vi "Wait-for-lasing-end.vi"(8 "error in (no error)":errorcluster, 11 "Object ref in":T1) -> (0 "error out":errorcluster, 1 "Succes?":bool, 3 "Object ref out":T1)   [LabVIEW 2013, in "SLMControl.lvlib" / "SC-Main.lvclass"]
uses:
  SC-Main.lvclass
  Object-reference.ctl
  UI/Control-names.ctl
  SC-Main.lvclass/SC-Main.ctl
  Read Lasing control.vi
  Read UI.vi
  UI/Set-control-boolean.vi
  UI/Set-control-string.vi
  UI/Set-control-double.vi
  SM1000/SM1000.lvclass
  UI/SC-UI.lvclass
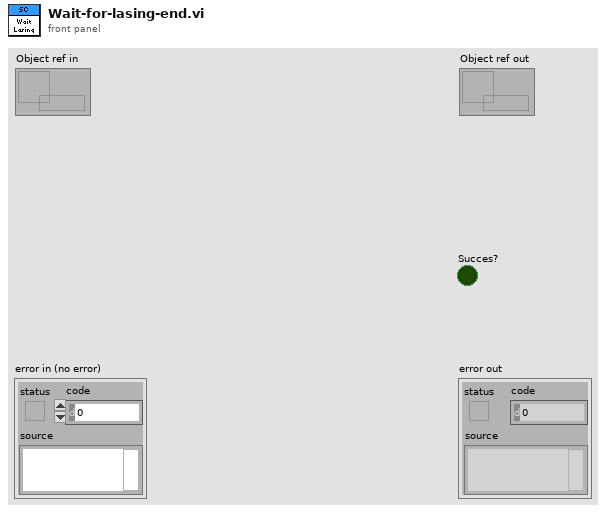
[diagram p1: front panel]
types:
  T1 = typedef "SLMControl.lvlib/SC-Main.lvclass/Object-reference.ctl" = refnum<data-value>
  T2 = typedef "SLMControl.lvlib/SC-UI.lvclass/Control-names.ctl" = enum16{"Com-in", "Com-out", "Help", "Status", "Load configuration", "Save configuration", "Load lasing files", "Load deposition files", "Clear", "Files", "Activate", "Execute", "Abort", "Options", "Current layer", "Current iteration", "Last elapsed time", "Deposition status", "Lasing job", "Status LEDs", "Exiting led", "Initialized led", "Files loaded led", "Activated led", "Executing led", "Deposition led", "Lasing job led", "Lasing led"}
  T3 = typedef "SLMControl.lvlib/SM1000.lvclass/Object-reference.ctl" = refnum<data-value>
  T4 = typedef "SLMControl.lvlib/SC-UI.lvclass/Panes-reference.ctl" = refnum<data-value>
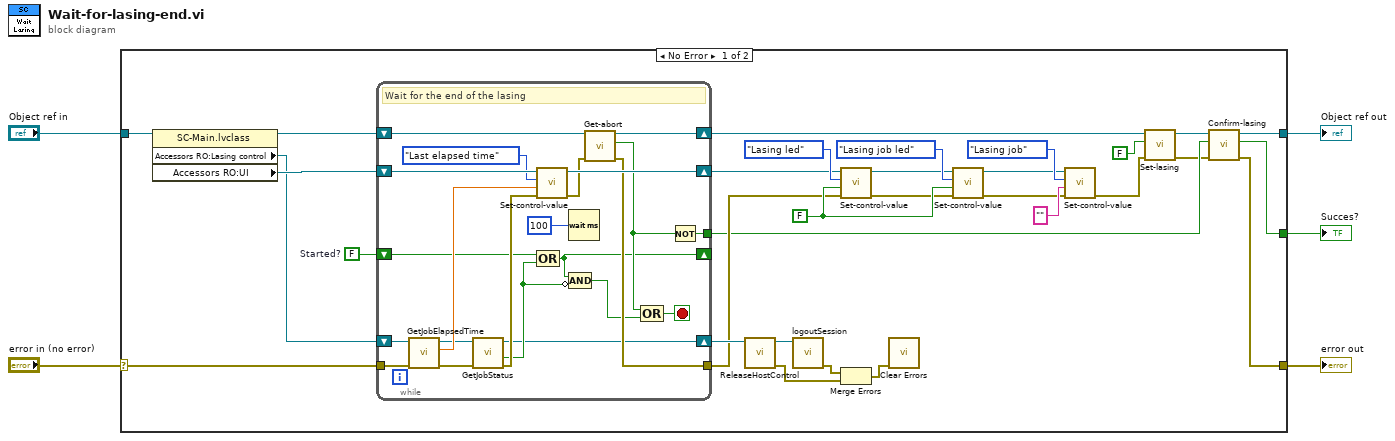
[diagram p0: block diagram]
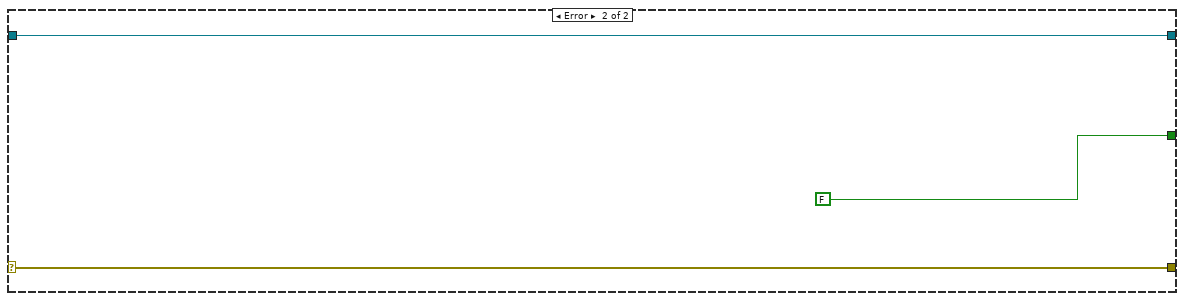
[diagram p2: hidden frame]
diagram:
  n1 = case shown="No Error" "error in (no error)" {
    selector: "error in (no error)" -> [w19 w61]
    tunnel: [w7 w61] -> w4
    tunnel: [w10 w60] -> w2
    tunnel: "Object ref in" -> [w36 w60]
    tunnel: [w9 FALSE] -> w1
    frame No Error {
      w12 = FALSE  # Started?
      w27 = FALSE
      n2 = property class="SC-Main.lvclass"(reference=w36) -> (reference out=w35:T1, "Accessors RO:Lasing control"=w13:T3, "Accessors RO:UI"=w34:T4)  [unwired: 1 in, 1 out]
      n3 = while {
        shift-right: [w51] -> w23
        shift-left: w35 -> [w58]
        tunnel: [w56] -> w8
        shift-right: [w40] -> w20
        shift-left: w13 -> [w39]
        tunnel: [w49] -> w18
        shift-right: [w54] -> w30
        shift-left: w34 -> [w55]
        tunnel: w19 -> [w38]
        shift-right: [w42] -> _
        shift-left: w12 -> [w44]
        stop <- w57 stop-if-true
        # "Wait for the end of the lasing"
        n4 = call "GetJobElapsedTime.vi"("error in (no error)"=w38, "SM1000-control in"=w39) -> ("error out"=w46:errorcluster, "Elapsed time"=w52:dbl, "SM1000-control out"=w37:T3)  [unwired: 7 in]
        n5 = call "GetJobStatus.vi"("error in (no error)"=w46, "SM1000-control in"=w37) -> ("error out"=w45:errorcluster, "Busy?"=w43:bool, "SM1000-control out"=w40:T3)  [unwired: 7 in]
        n6 = call-poly "Set-control-value.vi"("error in (no error)"=w45, "Value"=w52, "Control name"=Control-names."Last elapsed time", "Panes in"=w55) -> ("error out"=w50:errorcluster, "Panes out"=w54:T4)  [unwired: 6 in]
        n7 = Compound Arithmetic op=OR(w44, w43) -> (w42:bool)
        n8 = Wait (ms)(milliseconds to wait=u32 100) -> ()  [unwired: 1 out]
        n9 = Compound Arithmetic op=AND(w42, invert w43) -> (w41:bool)
        n10 = call "Get-abort.vi"("error in (no error)"=w50, "Object ref in"=w58) -> ("error out"=w49:errorcluster, "Abort"=w48:bool, "Object ref out"=w51:T1)  [unwired: 7 in]
        n11 = Compound Arithmetic op=OR(w48, w41) -> (w57:bool)
        n12 = Not(x=w48) -> (.not. x?=w56:bool)
      }
      n13 = call "ReleaseHostControl.vi"("SM1000-control in"=w20) -> ("error out"=w15:errorcluster, "SM1000-control out"=w17:T3)  [unwired: 9 in]
      n14 = call "logoutSession.vi"("SM1000-control in"=w17) -> ("error out"=w16:errorcluster)  [unwired: 9 in, 1 out]
      n15 = call-poly "Set-control-value.vi"("error in (no error)"=w18, "Value"=w27, "Control name"=Control-names."Lasing led", "Panes in"=w30) -> ("error out"=w25:errorcluster, "Panes out"=w29:T4)  [unwired: 6 in]
      n16 = Merge Errors(w16, w15) -> (w14:errorcluster)
      n17 = call <vilib>:"Clear Errors.vi"("error in (no error)"=w14) -> ()  [unwired: 6 in, 1 out]
      n18 = call-poly "Set-control-value.vi"("error in (no error)"=w25, "Value"=w27, "Control name"=Control-names."Lasing job led", "Panes in"=w29) -> ("error out"=w24:errorcluster, "Panes out"=w28:T4)  [unwired: 6 in]
      n19 = call-poly "Set-control-value.vi"("error in (no error)"=w24, "Value"="", "Control name"=Control-names."Lasing job", "Panes in"=w28) -> ("error out"=w22:errorcluster)  [unwired: 6 in, 1 out]
      n20 = call "Set-lasing.vi"("error in (no error)"=w22, "Lasing?"=FALSE, "Object ref in"=w23) -> ("error out"=w6:errorcluster, "Object ref out"=w11:T1)  [unwired: 7 in]
      n21 = call "Confirm-lasing.vi"("error in (no error)"=w6, "Succes? in"=w8, "Data Value Reference in"=w11) -> ("error out"=w7:errorcluster, "Succes?"=w9:bool, "Data Value Reference out"=w10:T1)  [unwired: 6 in]
    }
    frame Error {
    }
  }
  "error out" <- w4
  "Object ref out" <- w2
  "Succes?" <- w1
